vi "Switch Solenoid.vi"(8 "error in (no error)":errorcluster, 11 "Feeder Actor.lvlib:Solenoid.lvclass":refnum<class "Solenoid.lvclass">) -> (0 "error out":errorcluster, 3 "Actor out":refnum<class "Actor.lvclass">)   [LabVIEW 2018, in "Feeder Actor.lvlib" / "Solenoid.lvclass"]
uses:
  Solenoid.lvclass
  C:/Program Files/National Instruments/LabVIEW 2018/vi.lib/ActorFramework/Actor/Actor.lvclass
  <vilib>/ActorFramework/Actor/Actor.lvclass
  Solenoid.lvclass/Solenoid.ctl
  <vilib>/DAQmx/write.llb/DAQmx Write (Digital Bool 1Line 1Point).vi
  <vilib>/DAQmx/miscellaneous.llb/DAQmx Fill In Error Info.vi
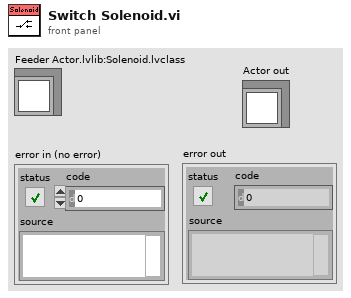
[diagram p1: front panel]
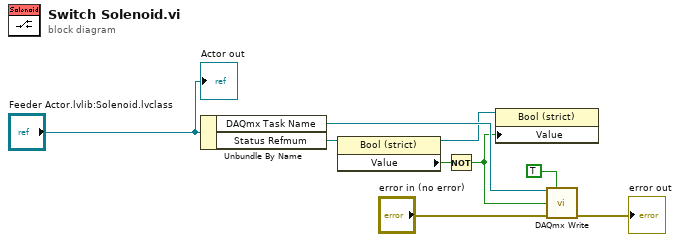
[diagram p0: block diagram]
diagram:
  n1 = Unbundle By Name("Feeder Actor.lvlib:Solenoid.lvclass") -> ("DAQmx Task Name"=w7:refnum<k21>, "Status Refmum"=w6:refnum<vi>)
  n2 = property class="Bool (strict)"(reference=w6) -> (reference out=w4:refnum<vi>, "Value"=w3:bool)  [unwired: 1 in, 1 out]
  n3 = Not(x=w3) -> (.not. x?=w1:bool)
  n4 = property class="Bool (strict)"(reference=w4, "Value"=w1) -> ()  [unwired: 1 in, 2 out]
  n5 = call-poly <vilib>:"DAQmx Write.vi"("task/channels in"=w7, "auto start"=TRUE, "data"=w1, "error in"="error in (no error)") -> ("error out"=→"error out":errorcluster)  [unwired: 9 in, 2 out]
  "Actor out" <- "Feeder Actor.lvlib:Solenoid.lvclass"
